vi "tcp_init.vi"(11 "port":u16=9150) -> (0 "error out":errorcluster, 3 "output cluster":T1)   [LabVIEW 2018]
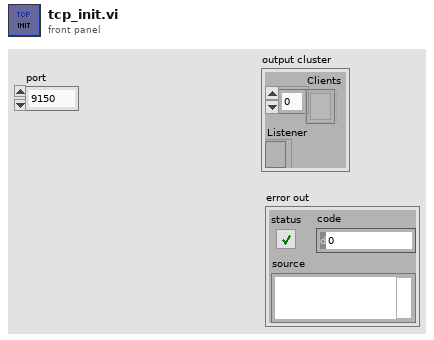
[diagram p1: front panel]
types:
  T1 = cluster{"Clients":refnum<k5>[], "Listener":refnum<k5>}
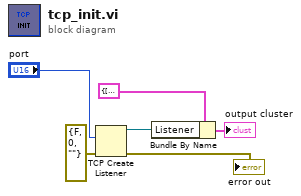
[diagram p0: block diagram]
diagram:
  n1 = TCP Create Listener(8:errorcluster {"status"=FALSE, "code"=0, "source"=""} ("error in (no error)"), 10:"port") -> (0:→"error out":errorcluster, 3:w6:refnum<k5>)  [unwired: 4 out]
  n2 = Bundle By Name(cluster=T1 {"Clients"=[], "Listener"=refnum} ("Data"), "Listener"=w6) -> (→"output cluster":T1)
